vi "Wait Event.vi"(8 "error in (no error)":errorcluster, 9 "timeout (-1)":dbl[unit]=-0.001, 10 "wait event":T1=2 items=["install"=2, "remove"=3]) -> (0 "error out":errorcluster, 2 "return value":i32)   [LabVIEW 2017, in "HighFinesse WS5.lvlib"]
doc: "Installs or removes a wait event, which is necessary before checking for changes in the WLM."
uses:
  HighFinesse WS5.lvlib
  Control typedefs.llb/Wait Event.ctl
  <vilib>/Utility/error.llb/DialogType.ctl
  wlmData.dll
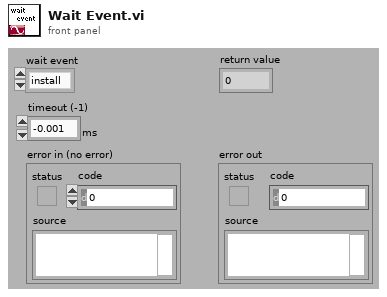
[diagram p1: front panel]
types:
  T1 = typedef "HighFinesse WS5.lvlib/Wait Event.ctl" = i32
  T2 = typedef "DialogType.ctl" = u16
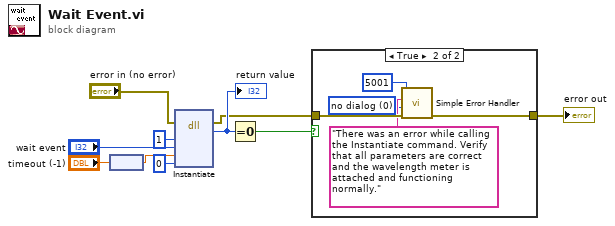
[diagram p0: block diagram]
diagram:
  n1 = node("timeout (-1)") -> (w1:dbl)
  n2 = dll-call lib="C:/LabVIEW-programs/Instruments/Wavelength meter/HighFinesse WS5/wlmData.dll" fn="Instantiate"(error in="error in (no error)", "RFC"=1, "Mode"="wait event", "P1"=w1, "P2"=0) -> (error out=w5:errorcluster, "return type"=w6:i32)  [unwired: 5 in, 2 out]
  "return value" <- w6
  n3 = Equal To 0?(x=w6) -> (x = 0?=w7:bool)
  n4 = case shown="True" w7 {
    tunnel: w5 -> [w11 w16]
    tunnel: [w11 w13] -> w4
    frame False {
    }
    frame True {
      w14 = T2 0 items=["no dialog", "OK message", "continue or stop message", "OK message + warnings", "continue/stop + warnings"] ("type of dialog (OK msg:1)")
      n5 = call <vilib>:"Simple Error Handler.vi"("error code (no error:0)"=5001, "error source (\" \")"="There was an error while calling the Instantiate command. Verify that all parameters are correct and the wavelength meter is attached and functioning normally." ("error source (\" \")"), "type of dialog (OK msg:1)"=w14, "error in (no error)"=w16) -> ("error out"=w13:errorcluster)  [unwired: 5 out]
    }
  }
  "error out" <- w4
